vi "5.vi"() -> ()   [LabVIEW 2020]
panel:
  in  "Array":string[](array[string])
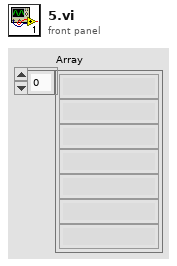
[diagram p1: front panel]
types:
  T1 = enum16{"open", "replace", "create", "open or create", "replace or create", "replace or create with confirmation"}
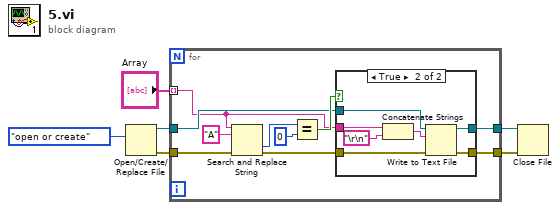
[diagram p0: block diagram]
diagram:
  n1 = Open/Create/Replace File(operation (0:open)=T1."open or create") -> (refnum out=w5:refnum<file>, error out=w3:errorcluster)  [unwired: 5 in, 1 out]
  n2 = for {
    tunnel: w5 -> [w10]
    tunnel: "Array" -> [w7] mode=indexing
    tunnel: w3 -> [w13]
    tunnel: [w8] -> w2
    tunnel: [w9] -> w1
    n3 = Search and Replace String(input string=w7, search string="A", error in=w13) -> (offset past replacement=w15:i32, error out=w11:errorcluster)  [unwired: 5 in, 2 out]
    n4 = Equal?(x=w15, y=0) -> (x = y?=w12:bool)
    n5 = case shown="True" w12 {
      tunnel: w11 -> [w18 w25]
      tunnel: w10 -> [w17 w24]
      tunnel: [w18 w23] -> w9
      tunnel: [w17 w22] -> w8
      tunnel: w7 -> [_ w21]
      frame False {
      }
      frame True {
        n6 = Concatenate Strings(w21, "\r\n") -> (w19:string)
        n7 = Write to Text File(file (use dialog)=w24, text=w19, error in=w25) -> (refnum out=w22:refnum<file>, error out=w23:errorcluster)  [unwired: 1 in, 1 out]
      }
    }
  }
  n8 = Close File(refnum=w2, error in=w1) -> ()  [unwired: 2 out]
